vi "Receive vi.vi"() -> ()   [LabVIEW 2014]
panel:
  out "TC03":dbl
  in  "클러스터":T1
  out "데이터 출력 2":dbl
  out "데이터 출력":dbl
  in  "정지":bool
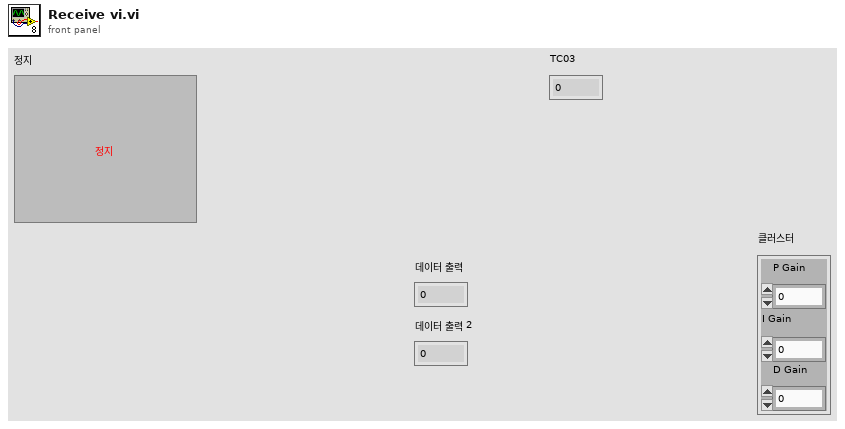
[diagram p1: front panel]
types:
  T1 = cluster{"P Gain":dbl, "I Gain":dbl, "D Gain":dbl}
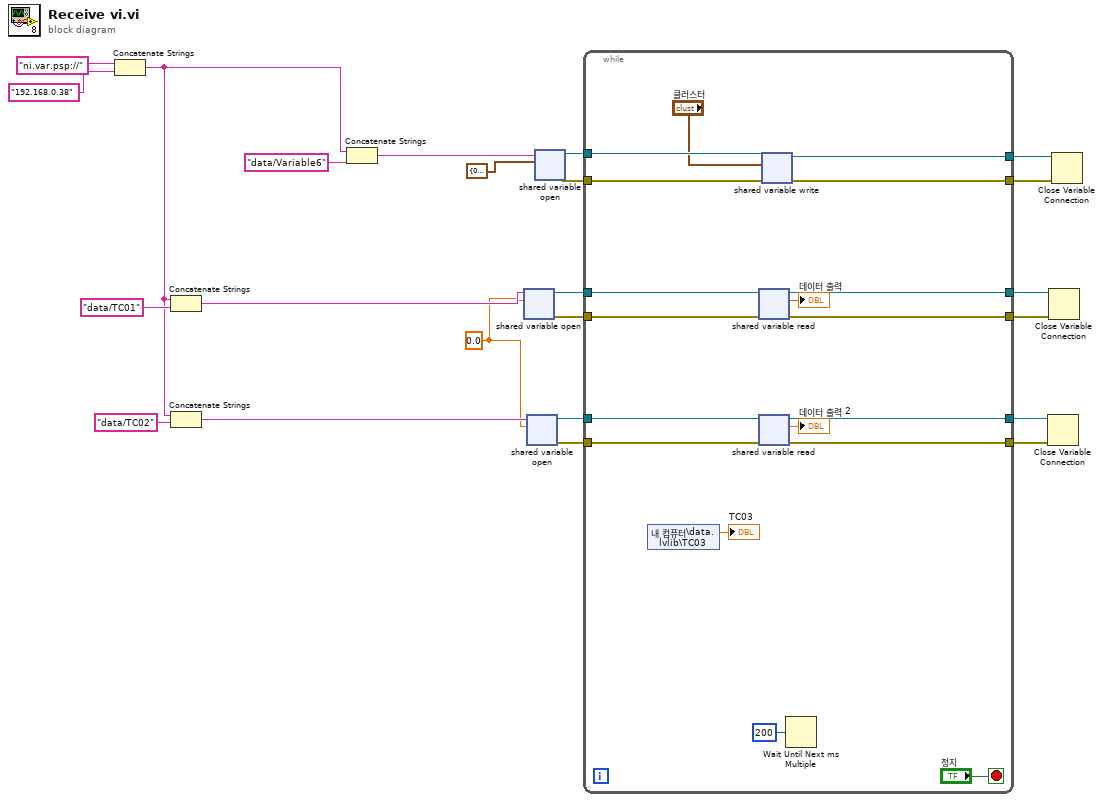
[diagram p0: block diagram]
diagram:
  w1 = 0.0
  n1 = Concatenate Strings("ni.var.psp://", "192.168.0.38" ("문자열")) -> (w4:string)
  n2 = Concatenate Strings(w4, "data/TC01") -> (w9:string)
  n3 = Concatenate Strings(w4, "data/TC02") -> (w6:string)
  n4 = Concatenate Strings(w4, "data/Variable6") -> (w5:string)
  n5 = shared-variable-open(w9, w1) -> (w23:refnum<k21>, w20:errorcluster)  [unwired: 2 in]
  n6 = shared-variable-open(w6, w1) -> (w19:refnum<k21>, w18:errorcluster)  [unwired: 2 in]
  n7 = shared-variable-open(w5, T1 {"P Gain"=0.0, "I Gain"=0.0, "D Gain"=0.0} ("클러스터 2")) -> (w15:refnum<k21>, w14:errorcluster)  [unwired: 2 in]
  n8 = while {
    tunnel: w23 -> [w41]
    tunnel: [w40] -> w22
    tunnel: [w39] -> w21
    tunnel: w20 -> [w38]
    tunnel: w19 -> [w37]
    tunnel: w18 -> [w36]
    tunnel: [w35] -> w17
    tunnel: [w34] -> w16
    tunnel: w15 -> [w31]
    tunnel: w14 -> [w30]
    tunnel: [w29] -> w13
    tunnel: [w28] -> w12
    stop <- "정지" stop-if-true
    n9 = shared-variable "내 컴퓨터\\data.lvlib\\TC03"() -> (→"TC03":dbl)  [unwired: 1 in, 1 out]
    n10 = shared-variable-read(w41, w38) -> (w40:refnum<k21>, w39:errorcluster, →"데이터 출력":dbl)  [unwired: 1 out]
    n11 = shared-variable-read(w37, w36) -> (w34:refnum<k21>, w35:errorcluster, →"데이터 출력 2":dbl)  [unwired: 1 out]
    n12 = shared-variable-write(w31, w30, "클러스터") -> (w29:refnum<k21>, w28:errorcluster)
    n13 = Wait Until Next ms Multiple(millisecond multiple=u32 200 ("ms 배수")) -> ()  [unwired: 1 out]
  }
  n14 = Close Variable Connection(8:w17, 11:w16) -> ()  [unwired: 1 out]
  n15 = Close Variable Connection(8:w21, 11:w22) -> ()  [unwired: 1 out]
  n16 = Close Variable Connection(8:w12, 11:w13) -> ()  [unwired: 1 out]
